vi "mqttCmdAcknowledge.vi"(0 "mqttConnect in":refnum<class "mqttCmdConnect.lvclass">, 7 "mqtt in":refnum<class "mqtt.lvclass">, 11 "error in (no error)":errorcluster) -> (4 "mqttConnect out":refnum<class "mqttCmdConnect.lvclass">, 8 "notification":T1, 15 "error out":errorcluster)   [LabVIEW 2018, in "labview-mqtt.lvlib" / "mqttCmdConnect.lvclass"]
uses:
  mqttCmdConnect.lvclass
  D:/OneDrive/_WorkingOn/IECube/MQTT LabVIEW/mqtt-LabVIEW-master-yao/src/class/mqtt/mqttCmd/mqttCmd.lvclass
  mqttTypedef/mqttRXdataCluster.ctl
  mqttTypedef/mqttFixedHeaderResponse.ctl
  mqttTypedef/mqttQOSlevel.ctl
  mqttTypedef/mqttMessageType.ctl
  mqtt.lvclass
  mqttTypedef/mqttConnectionStatus.ctl
  mqttCmdConnect.lvclass/mqttCmdConnect.ctl
  mqttCmd.lvclass/mqttCmd.ctl
  labview-mqtt.lvlib
  mqttCmd.lvclass
panel:
  out "payload (HEX)":u8[](array[numeric]) format="%02x"
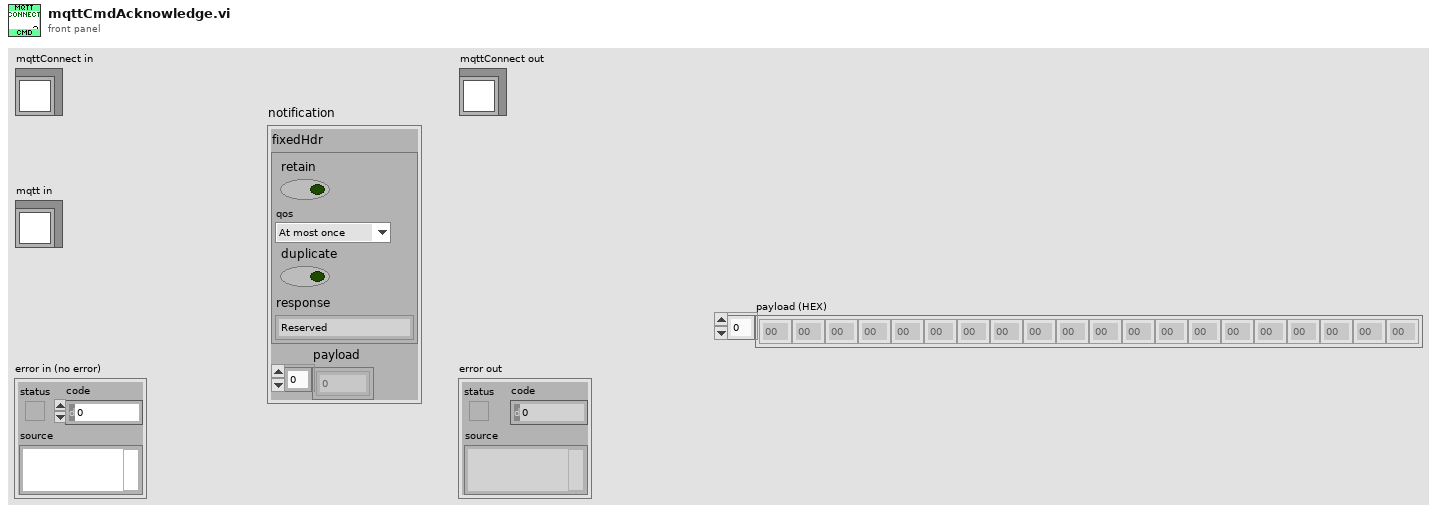
[diagram p1: front panel]
types:
  T1 = typedef "labview-mqtt.lvlib/mqttRXdataCluster.ctl" = cluster{"fixedHdr":T2, "payload":u8[]}
  T2 = typedef "labview-mqtt.lvlib/mqttFixedHeaderResponse.ctl" = cluster{"retain":bool, "qos":T3, "duplicate":bool, "response":T4}
  T3 = typedef "labview-mqtt.lvlib/mqttQOSlevel.ctl" = enum8{"At most once", "At least once", "Exactly once", "Reserved"}
  T4 = typedef "labview-mqtt.lvlib/mqttMessageType.ctl" = enum32{"Reserved", "CONNECT", "CONNACK", "PUBLISH", "PUBACK", "PUBREC", "PUBREL", "PUBCOMP", "SUBSCRIBE", "SUBACK", "UNSUBSCRIBE", "UNSUBACK", "PINGREQ", "PINGRESP", "DISCONNECT", "Reserved2"}
  T5 = typedef "labview-mqtt.lvlib/mqttConnectionStatus.ctl" = enum16{"Connection accepted", "Connection refused: unacceptable protocol version", "Connection refused: identifier rejected", "Connection refused: Server unavailable", "Connection refused: bad user name or password", "Connection refused: not authorized"}
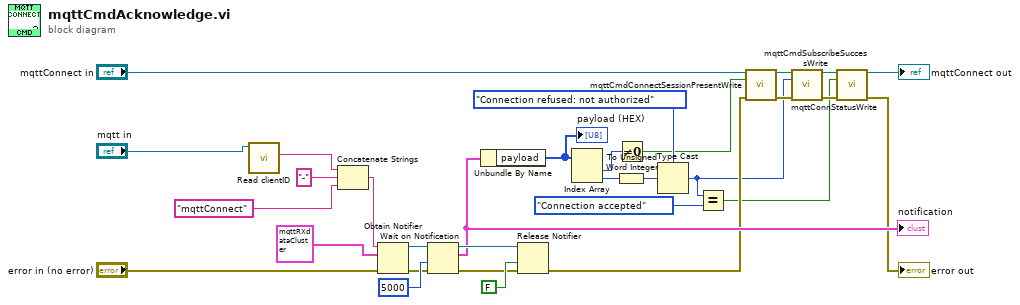
[diagram p0: block diagram]
diagram:
  n1 = call-dynamic "Read clientID.vi"("mqtt in"="mqtt in") -> ("clientID"=w3:string)  [unwired: 8 in, 2 out]
  n2 = Concatenate Strings(w3, "-" ("string"), "mqttConnect" ("name (unnamed)")) -> (w1:string)
  n3 = Obtain Notifier(name (unnamed)=w1, notification data type=T1 {"fixedHdr"={"retain"=FALSE, "qos"=enum."At most once", "duplicate"=FALSE, "response"=enum."Reserved"}, "payload"=[]} ("output cluster"), error in (no error)="error in (no error)") -> (notifier out=w27:refnum<notifier>, error out=w26:errorcluster)  [unwired: 1 in, 1 out]
  n4 = Wait on Notification(notifier=w27, timeout in ms (-1)=5000, error in (no error)=w26) -> (notifier out=w30:refnum<notifier>, notification=w19:T1, error out=w29:errorcluster)  [unwired: 1 in, 1 out]
  "notification" <- w19
  n5 = Unbundle By Name(w19) -> ("payload"=w18:u8[])
  "payload (HEX)" <- w18
  n6 = Release Notifier(notifier=w30, force destroy? (F)=FALSE, error in (no error)=w29) -> (error out=w14:errorcluster)  [unwired: 2 out]
  n7 = Index Array(array=w18) -> (element #1=w23:u8, element #2=w21:u8)  [unwired: 2 in]
  n8 = To Unsigned Word Integer(number=w21) -> (unsigned 16bit integer=w20:u16)
  n9 = Not Equal To 0?(x=w23) -> (x != 0?=w17:bool)
  n10 = Type Cast(type=mqttConnectionStatus."Connection refused: not authorized" ("connStatus"), x=w20) -> (*(type *) &x=w7:T5)
  n11 = Equal?(x=w7, y=mqttConnectionStatus."Connection accepted") -> (x = y?=w6:bool)
  n12 = call "mqttCmdConnectSessionPresentWrite.vi"("mqttConnect in"="mqttConnect in", "sessionPresent"=w17, "error in (no error)"=w14) -> ("mqttConnect out"=w15:refnum<class "mqttCmdConnect.lvclass">, "error out"=w13:errorcluster)  [unwired: 11 in]
  n13 = call "mqttConnStatusWrite.vi"("mqttConnect in"=w15, "connStatus"=w7, "error in (no error)"=w13) -> ("mqttConnect out"=w12:refnum<class "mqttCmdConnect.lvclass">, "error out"=w9:errorcluster)  [unwired: 11 in]
  n14 = call "mqttCmdSubscribeSuccessWrite.vi"("mqttBrokerCommand in"=w12, "success"=w6, "error in (no error)"=w9) -> ("mqttBrokerCommand out"=→"mqttConnect out":refnum<class "mqttCmdConnect.lvclass">, "error out"=→"error out":errorcluster)  [unwired: 11 in]
